vi "Net DC Global Gain Trim.vi"(0 "15mA_Offset":dbl=1.0, 1 "10mA_Offset":dbl=1.0, 2 "5mA_Offset":dbl=1.0, 3 "2mA_Offset":dbl=1.0) -> (5 "Global Gain Correction out":dbl)   [LabVIEW 2010]
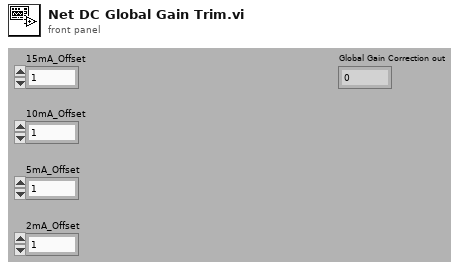
[diagram p1: front panel]
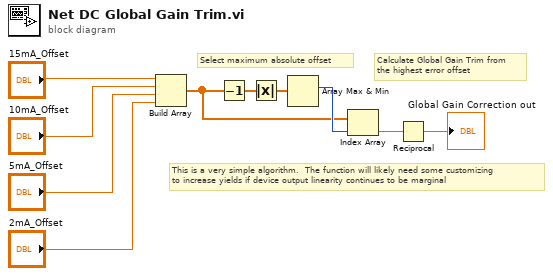
[diagram p0: block diagram]
diagram:
  # "This is a very simple algorithm.  The function will likely need some customizing \nto increase yields if device output linearity continues to be marginal"
  # "Calculate Global Gain Trim from\nthe highest error offset"
  # "Select maximum absolute offset"
  n1 = Build Array("15mA_Offset", "10mA_Offset", "5mA_Offset", "2mA_Offset") -> (w3:dbl[])
  n2 = Decrement(x=w3) -> (x-1=w4:dbl[])
  n3 = Absolute Value(x=w4) -> (abs(x)=w6:dbl[])
  n4 = Array Max & Min(array=w6) -> (max index (indices)=w5:i32)  [unwired: 3 out]
  n5 = Index Array(array=w3, index=w5) -> (element=w2:dbl)
  n6 = Reciprocal(x=w2) -> (1/x=→"Global Gain Correction out":dbl)
